vi "Socket_Write EOLData.vi"(8 "data in":string[](array[string]), 11 "station name":string) -> ()   [LabVIEW 2018]
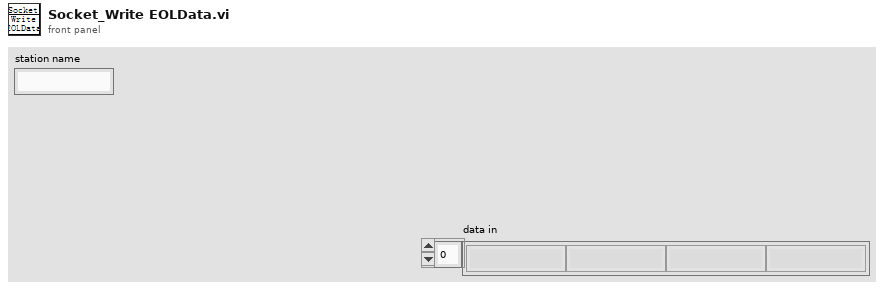
[diagram p1: front panel]
types:
  T1 = enum16{"Read", "Write", "ReadWrite", "BufferedRead", "BufferedReadWrite"}
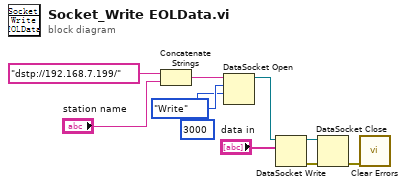
[diagram p0: block diagram]
diagram:
  n1 = Concatenate Strings("dstp://192.168.7.199/" ("URL"), "station name") -> (w7:string)
  n2 = DataSocket Open(9:3000 ("毫秒超时(10000)"), 10:T1."Write" ("模式"), 11:w7) -> (3:w6:refnum<k13>)  [unwired: 1 in, 1 out]
  n3 = DataSocket Write(10:"data in", 11:w6) -> (0:w3:errorcluster, 3:w4:refnum<k13>)  [unwired: 2 in, 1 out]
  n4 = DataSocket Close(8:w3, 11:w4) -> (0:w2:errorcluster)  [unwired: 1 in, 1 out]
  n5 = call <vilib>:"Clear Errors.vi"("error in (no error)"=w2) -> ()  [unwired: 5 in, 2 out]
